vi "Engine-Throttle-TB2.vi"(8 "Error In":errorcluster, 11 "DSI Reference":refnum<class "DCM-DSI.lvclass">) -> (0 "Error Out":errorcluster, 3 "DSI Reference":refnum<class "DCM-DSI.lvclass">)   [LabVIEW 2016, in "DSI-RT.lvlib"]
uses:
  DSI-RT.lvlib
  Classes/DCM-DSI/DCM-DSI.lvclass
  <vilib>/Powertrain Controls/Device Drivers/DCM/HH/RT/Setup.ctl
  <vilib>/Powertrain Controls/Device Drivers/DCM/HH/FPGA/Mode.ctl
  <vilib>/Powertrain Controls/Device Drivers/DCM/Rev0/FPGA/Digital Channel.ctl
  <vilib>/Powertrain Controls/Device Drivers/DCM/HH/RT/Angle Control.ctl
  <vilib>/Powertrain Controls/Device Drivers/DCM/Rev0/RT/DCM - RT.lvclass/DCM - RT.ctl
  <vilib>/Powertrain Controls/Device Drivers/DCM/HH/RT/Mode.ctl
  <vilib>/Powertrain Controls/Device Drivers/DCM/Rev0/RT/Read HH Mode.vi
  Classes/DCM-DSI/Read HH Command.vi
  Classes/DCM-DSI/Read dt.vi
  Classes/DCM-DSI/Read HH Status.vi
  Classes/DCM-DSI/Read System ADC.vi
  Classes/DCM-DSI/Read Channels.vi
  Classes/DCM-DSI/Read DCM Ref.vi
  <vilib>/Powertrain Controls/Device Drivers/Tools/Real-Time/ticks2time.vi
  Classes/DCM-DSI/Write HH Command.vi
  <vilib>/Powertrain Controls/Device Drivers/DCM/Rev0/RT/DCM - RT.lvclass
  <vilib>/addons/Software Calibration Management/xSCM/CalPoint.xnode
  <vilib>/Powertrain Controls/Device Drivers/DCM/HH/RT/DCM - RT - HH.lvlib
  <vilib>/Powertrain Controls/Device Drivers/DCM/Rev0/FPGA/DCM - FPGA.lvlib
  <vilib>/Powertrain Controls/Device Drivers/DCM/HH/FPGA/DCM - FPGA - HH.lvlib
  <vilib>/addons/Software Calibration Management/xSCM/ni_scm.dll
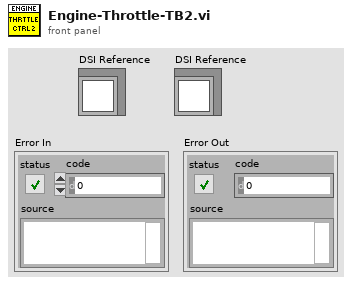
[diagram p1: front panel]
types:
  T1 = typedef "DCM - FPGA - HH.lvlib/Mode.ctl" = enum8{"Off", "Direct", "Pulse Width Modulation", "Engine Position Tracking"}
  T2 = cluster{"ModulePresent":bool, "H1Sense (A)":sgl, "H2Sense (A)":sgl, "Analog1 (V)":sgl, "Analog2 (V)":sgl, "Battery (V)":sgl, "Temperature (C)":sgl, "H1Fault":bool, "H2Fault":bool}
  T3 = typedef "DCM - RT - HH.lvlib/Setup.ctl" = cluster{"Mode":T1, "Digital Input":T4, "Polarity":bool, "Frequency [Hz]":sgl, "Duty Cycle [%]":sgl, "TDC Offset [CAD]":sgl, "Window Start [DBTDC]":sgl, "Window End [DBTDC]":sgl, "Angles":T5[], "Skip Fire":bool, "Skip Fire Index":u8}
  T4 = typedef "DCM - FPGA.lvlib/Digital Channel.ctl" = enum8{"Unused", "User OS", "Diff IO 1", "Diff IO 2", "Diff IO 3", "Diff IO 4", "Diff IO 5", "Diff IO 6", "Diff IO 7", "Diff IO 8", "Aux 1", "Aux 2", "Aux 3", "Aux 4", "Aux 5", "Aux 6", "Aux 7", "Aux 8", "Aux 9", "Aux 10", "Aux 11", "Aux 12", "Aux 13", "Aux 14", "Aux 15", "Aux 16"}
  T5 = typedef "DCM - RT - HH.lvlib/Angle Control.ctl" = cluster{"Enable":bool, "Location [DBTDC]":sgl, "Duration [s]":sgl}
  T6 = typedef "DCM - RT - HH.lvlib/Status.ctl" = cluster{"Current [A]":sgl, "Config Error":bool, "Short Fault":bool, "Open Fault":bool, "Period Min [A]":sgl, "Period Max [A]":sgl, "Period Avg [A]":sgl, "On Avg [A]":sgl}
  T7 = typedef "DCM - RT.lvclass/System ADC.ctl" = cluster{"AI 1 [V]":sgl, "AI 2 [V]":sgl, "AI 3 [V]":sgl, "AI 4 [V]":sgl, "AI 5 [V]":sgl, "AI 6 [V]":sgl, "AI 7 [V]":sgl, "AI 8 [V]":sgl, "AI 9 [V]":sgl, "AI 10 [V]":sgl, "AI 11 [V]":sgl, "AI 12 [V]":sgl, "Temp HH 1-6 [C]":sgl, "Temp HH 7-12 [C]":sgl, "Temp DI A [C]":sgl, "Temp DI Zener A [C]":sgl, "Temp DI B [C]":sgl, "Temp DI Zener B [C]":sgl, "Temp CPU [C]":sgl, "Temp Fan Intake [C]":sgl, "Temp Secondary A [C]":sgl, "Temp Primary A [C]":sgl, "Temp Boost B [C]":sgl, "Primary Range [V]":sgl, "Primary A1A2 [V]":sgl, "Primary A3A4 [V]":sgl, "Primary B3B4 [V]":sgl, "Primary B1B2 [V]":sgl, "Secondary A1A2 [V]":sgl, "Secondary A3A4 [V]":sgl, "Secondary B3B4 [V]":sgl, "Secondary B1B2 [V]":sgl, "Ext HV A [V]":sgl, "Ext HV B [V]":sgl, "FET Driver [V]":sgl, "Fan [V]":sgl, "Battery [V]":sgl, "DRVP [V]":sgl, "Key [V]":sgl, "DI Zener A [V]":sgl, "DI Zener B [V]":sgl, "Pump Zener A [V]":sgl, "Pump Zener B [V]":sgl, "MPRD [V]":sgl}
  T8 = typedef "DCM-DSI.lvclass/Channel.ctl" = cluster{"Name":string, "Unit":string, "Value":sgl}
  T9 = typedef "DCM - RT - HH.lvlib/Mode.ctl" = enum16{"Off", "Lowside", "Highside", "PFI", "Full H", "3-Phase"}
  T10 = cluster{"Analog1 Range [V]":sgl[], "Analog2 Range [V]":sgl[], "Position Range":sgl[]}
  T11 = cluster{"TLead [sec]":sgl, "TLag [sec]":sgl, "KRpos [V/ ]":sgl, "TIpos [sec]":sgl, "TDpos [sec]":sgl, "KRneg [V/ ]":sgl, "TIneg [sec]":sgl, "TDneg [sec]":sgl, "LH Position Band":sgl, "U LH (V)":sgl, "U LH Lag [sec]":sgl, "US (V)":sgl, "US Lag [sec]":sgl, "LH Position":sgl, "Motor Resistance [Ohms]":sgl, "Position Fault Thresh":sgl}
  T12 = cluster{"Pos Cal Init Delay (sec)":sgl, "Pos Cal Return From Positive Delay (sec)":sgl, "Pos Cal Return From Negative Delay (sec)":sgl, "u Pos Cal Positive Init (V)":sgl, "u Pos Cal Negative Init (V)":sgl, "u Pos Cal Inc (V)":sgl, "u Pos Cal Dec (V)":sgl, "u Pos Cal Inc Thresh (V)":sgl, "u Pos Cal Dec Thresh (V)":sgl, "Pos Cal Offset (V)":sgl, "Pos Cal Diff Thresh (V)":sgl}
  T13 = enum16{"IDLE", "POSITION CALIBRATION", "CONTROL CALIBRATION", "CONTROL"}
  T14 = cluster{"Primary Analog Range (V)":sgl[], "Secondary Analog Range (V)":sgl[], "Position Range":sgl[], "Position Calibrated":bool, "u Pos Cal Positive (V)":sgl, "u Pos Cal Negative (V)":sgl, "u Limit Positive":bool, "u Limit Negative":bool, "Pos Cal Diff Fault":bool}
  T15 = typedef "Mode Status.ctl" = enum16{"IDLE", "POSITION CALIBRATION", "CONTROL CALIBRATION", "CONTROL"}
  T16 = cluster{"Primary Position":sgl, "Secondary Position":sgl, "AboveLH?":bool, "Position Fault":bool, "u Limit?":bool, "uLHc (V)":sgl, "uFc (V)":sgl, "uPID (V)":sgl, "u (V)":sgl}
  T17 = cluster{"Primary Analog Range (V)":sgl[], "Secondary Analog Range (V)":sgl[], "Position Range":sgl[]}
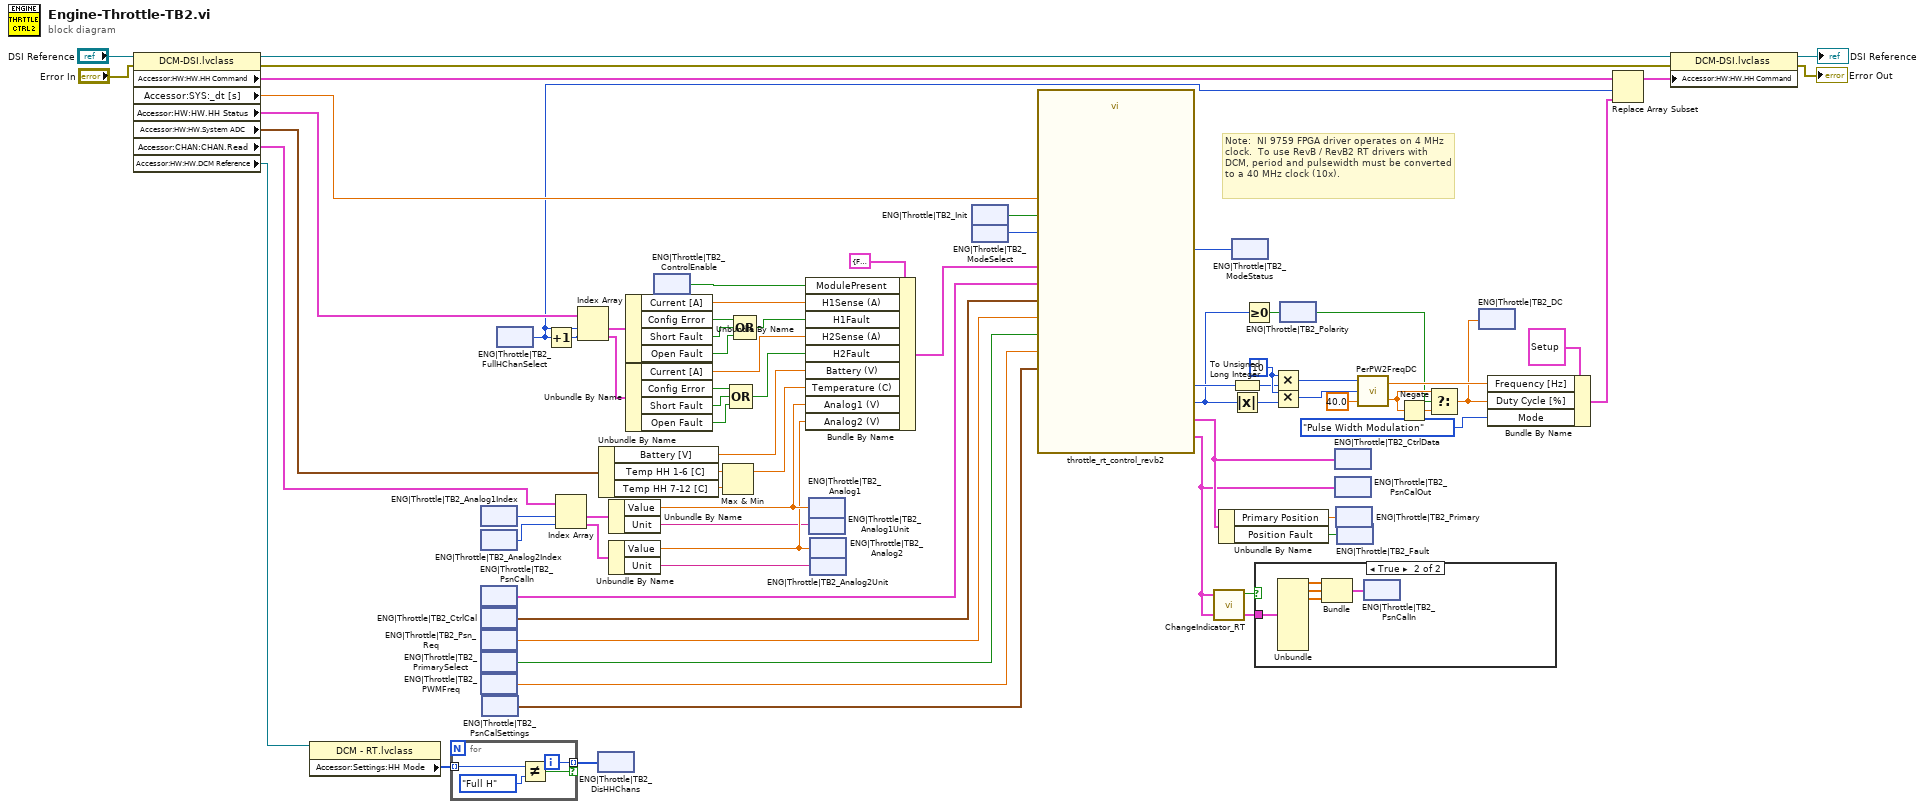
[diagram p0: block diagram]
diagram:
  w47 = u32 10 ("x")
  # "Note:  NI 9759 FPGA driver operates on 4 MHz clock.  To use RevB / RevB2 RT drivers with DCM, period and pulsewidth must be converted to a 40 MHz clock (10x)."
  n1 = property class="DCM-DSI.lvclass"(reference="DSI Reference", error in="Error In") -> (reference out=w29:refnum<class "DCM-DSI.lvclass">, error out=w28:errorcluster, "Accessor:HW:HW.HH Command"=w9:T3[], "Accessor:SYS:_dt [s]"=w10:sgl, "Accessor:HW:HW.HH Status"=w21:T6[], "Accessor:HW:HW.System ADC"=w22:T7, "Accessor:CHAN:CHAN.Read"=w23:T8[], "Accessor:HW:HW.DCM Reference"=w3:refnum<class "DCM - RT.lvclass">)
  n2 = property class="DCM - RT.lvclass"(reference=w3) -> ("Accessor:Settings:HH Mode"=w5:T9[])  [unwired: 1 in, 2 out]
  n3 = for {
    tunnel: [w77] -> w4 mode=indexing if=w76
    tunnel: w5 -> [w75] mode=indexing
    i -> [w77]
    n4 = Not Equal?(x=w75, y=Mode."Full H" ("Mode")) -> (x != y?=w76:bool)
  }
  n5 = xnode "ENG|Throttle|TB2_Analog1Index"() -> ("Value"=w74:i32)
  n6 = xnode "ENG|Throttle|TB2_Analog2Index"() -> ("Value"=w56:i32)
  n7 = xnode "ENG|Throttle|TB2_PsnCalIn"() -> ("Value"=w18:T10)
  n8 = xnode "ENG|Throttle|TB2_CtrlCal"() -> ("Value"=w17:T11)
  n9 = xnode "ENG|Throttle|TB2_Psn_Req"() -> ("Value"=w50:sgl)
  n10 = xnode "ENG|Throttle|TB2_PrimarySelect"() -> ("Value"=w45:bool)
  n11 = xnode "ENG|Throttle|TB2_PWMFreq"() -> ("Value"=w44:sgl)
  n12 = xnode "ENG|Throttle|TB2_PsnCalSettings"() -> ("Value"=w16:T12)
  n13 = xnode "ENG|Throttle|TB2_FullHChanSelect"() -> ("Value"=w6:i32)
  n14 = Increment(x=w6) -> (x+1=w43:i32)
  n15 = Index Array(array=w23, index #1=w74, index #2=w56) -> (element #1=w42:T8, element #2=w32:T8)
  n16 = Index Array(array=w21, index #1=w6, index #2=w43) -> (element #1=w68:T6, element #2=w67:T6)
  n17 = xnode "ENG|Throttle|TB2_DisHHChans"("Value"=w4) -> ()
  n18 = Unbundle By Name(w22) -> ("Battery [V]"=w54:sgl, "Temp HH 1-6 [C]"=w73:sgl, "Temp HH 7-12 [C]"=w72:sgl)
  n19 = Unbundle By Name(w42) -> ("Value"=w33:sgl, "Unit"=w15:string)
  n20 = Unbundle By Name(w32) -> ("Value"=w31:sgl, "Unit"=w14:string)
  n21 = Unbundle By Name(w68) -> ("Current [A]"=w66:sgl, "Config Error"=w64:bool, "Short Fault"=w63:bool, "Open Fault"=w62:bool)
  n22 = Unbundle By Name(w67) -> ("Current [A]"=w65:sgl, "Config Error"=w60:bool, "Short Fault"=w59:bool, "Open Fault"=w58:bool)
  n23 = xnode "ENG|Throttle|TB2_ControlEnable"() -> ("Value"=w40:bool)
  n24 = Max & Min(x=w73, y=w72) -> (max(x,y)=w55:sgl)  [unwired: 1 out]
  n25 = Compound Arithmetic op=OR(w60, w59, w58) -> (w57:bool)
  n26 = Compound Arithmetic op=OR(w64, w63, w62) -> (w61:bool)
  n27 = Bundle By Name(cluster=T2 {"ModulePresent"=FALSE, "H1Sense (A)"=0.0, "H2Sense (A)"=0.0, "Analog1 (V)"=0.0, "Analog2 (V)"=0.0, "Battery (V)"=0.0, "Temperature (C)"=0.0, "H1Fault"=FALSE, "H2Fault"=FALSE} ("ThrottleDataToControl"), "ModulePresent"=w40, "H1Sense (A)"=w66, "H1Fault"=w61, "H2Sense (A)"=w65, "H2Fault"=w57, "Battery (V)"=w54, "Temperature (C)"=w55, "Analog1 (V)"=w33, "Analog2 (V)"=w31) -> (w69:T2)
  n28 = xnode "ENG|Throttle|TB2_Analog1"("Value"=w33) -> ()
  n29 = xnode "ENG|Throttle|TB2_Analog1Unit"("Value"=w15) -> ()
  n30 = xnode "ENG|Throttle|TB2_Analog2"("Value"=w31) -> ()
  n31 = xnode "ENG|Throttle|TB2_Analog2Unit"("Value"=w14) -> ()
  n32 = xnode "ENG|Throttle|TB2_Init"() -> ("Value"=w39:bool)
  n33 = xnode "ENG|Throttle|TB2_ModeSelect"() -> ("Value"=w19:T13)
  n34 = call <vilib>:"throttle_rt_control_revb2.vi"("Mode Request"=w19, "Module Data"=w69, "Primary Position (F=1, T=2)"=w45, "PWM Frequency (Hz)"=w44, "Position Setpoint"=w50, "dt (sec)"=w10, "Position Cal Settings"=w16, "Position Cal In"=w18, "Control Cal In"=w17, "initialize"=w39) -> ("Position Cal Out"=w1:T14, "Mode Status"=w20:T15, "Control Data"=w11:T16, "Throttle Period Ticks"=w51:u16, "Throttle Pulse Width Ticks"=w49:i16)  [unwired: 4 in, 1 out]
  n35 = call "ChangeIndicator_RT.vi"("Input"=w1) -> ("Change"=w2:bool)  [unwired: 9 in]
  n36 = Unbundle By Name(w11) -> ("Primary Position"=w13:sgl, "Position Fault"=w12:bool)
  n37 = xnode "ENG|Throttle|TB2_ModeStatus"("Value"=w20) -> ()
  n38 = To Unsigned Long Integer(number=w51) -> (unsigned 32bit integer=w46:u32)
  n39 = Absolute Value(x=w49) -> (abs(x)=w48:i16)
  n40 = Greater Or Equal To 0?(x=w49) -> (x >= 0?=w35:bool)
  n41 = case shown="True" w2 {
    tunnel: w1 -> [_ w83]
    frame False {
    }
    frame True {
      n42 = Unbundle(w83) -> ("Primary Analog Range (V)"=w82:sgl[], "Secondary Analog Range (V)"=w81:sgl[], "Position Range"=w80:sgl[])  [unwired: 6 out]
      n43 = Bundle("Primary Analog Range (V)"=w82, "Secondary Analog Range (V)"=w81, "Position Range"=w80) -> (w79:T17)  [unwired: 1 in]
      n44 = xnode "ENG|Throttle|TB2_PsnCalIn"("Value"=w79) -> ()
    }
  }
  n45 = Multiply(x=w47, y=w46) -> (x*y=w53:u32)
  n46 = Multiply(x=w47, y=w48) -> (x*y=w52:u32)
  n47 = xnode "ENG|Throttle|TB2_Polarity"("Value"=w35) -> ()
  n48 = xnode "ENG|Throttle|TB2_CtrlData"("Value"=w11) -> ()
  n49 = xnode "ENG|Throttle|TB2_PsnCalOut"("Value"=w1) -> ()
  n50 = xnode "ENG|Throttle|TB2_Primary"("Value"=w13) -> ()
  n51 = xnode "ENG|Throttle|TB2_Fault"("Value"=w12) -> ()
  n52 = call <vilib>:"PerPW2FreqDC.vi"("Clock Frequency (MHz, 40)"=sgl 40.0, "PulseWidth(ticks)"=w52, "Period(ticks)"=w53) -> ("DutyCycle(%)"=w36:sgl, "Frequency(Hz)"=w41:sgl)
  n53 = Negate(x=w36) -> (-x=w37:sgl)
  n54 = Select(t=w36, s=w35, f=w37) -> (s? t:f=w38:sgl)
  n55 = xnode "ENG|Throttle|TB2_DC"("Value"=w38) -> ()
  n56 = Bundle By Name(cluster=T3 {"Mode"=enum."Off", "Digital Input"=enum."Unused", "Polarity"=FALSE, "Frequency [Hz]"=0.0, "Duty Cycle [%]"=0.0, "TDC Offset [CAD]"=0.0, "Window Start [DBTDC]"=0.0, "Window End [DBTDC]"=0.0, "Angles"=[{"Enable"=FALSE, "Location [DBTDC]"=0.0, "Duration [s]"=0.0}, {"Enable"=FALSE, "Location [DBTDC]"=0.0, "Duration [s]"=0.0}, {"Enable"=FALSE, "Location [DBTDC]"=0.0, "Duration [s]"=0.0}, {"Enable"=FALSE, "Location [DBTDC]"=0.0, "Duration [s]"=0.0}], "Skip Fire"=FALSE, "Skip Fire Index"=0} ("element"), "Frequency [Hz]"=w41, "Duty Cycle [%]"=w38, "Mode"=Mode."Pulse Width Modulation") -> (w7:T3)
  n57 = Replace Array Subset(array=w9, new element=w7, index=w6) -> (w8:T3[])
  n58 = property class="DCM-DSI.lvclass"(reference=w29, error in=w28, "Accessor:HW:HW.HH Command"=w8) -> (reference out=→"DSI Reference":refnum<class "DCM-DSI.lvclass">, error out=→"Error Out":errorcluster)
